vi "VIn SMU.vi"(8 "error in (no error)":errorcluster, 11 "Configuration":T2={"IVI Refnum in"="SMU4145", "Vin SMU Channel"="", "Voltage Level"=0.0, "Current Limit"=0.0}) -> (0 "error out":errorcluster, 3 "Measurements":T1)   [LabVIEW 2021]
uses:
  <instrlib>/niDCPower/nidcpower.llb/niDCPower Source Mode.ctl
  <instrlib>/niDCPower/nidcpower.llb/niDCPower Output Function.ctl
  controls/Current Meas.ctl
  controls/Data Holder.ctl
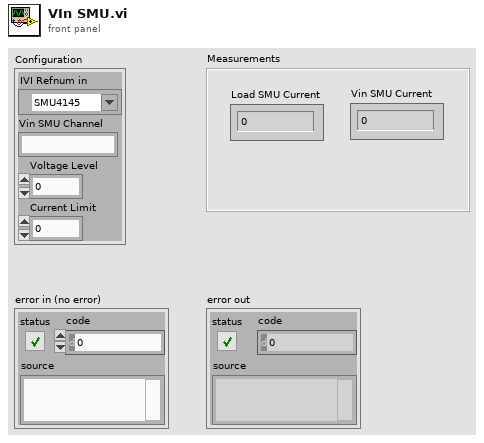
[diagram p1: front panel]
types:
  T1 = typedef "Current Meas.ctl" = cluster{"Load SMU Current":dbl, "Current Measurement":dbl}
  T2 = typedef "Data Holder.ctl" = cluster{"IVI Refnum in":refnum<k15>, "Vin SMU Channel":string, "Voltage Level":dbl, "Current Limit":dbl}
  T3 = typedef "niDCPower Output Function.ctl" = i32
  T4 = typedef "niDCPower Source Mode.ctl" = i32
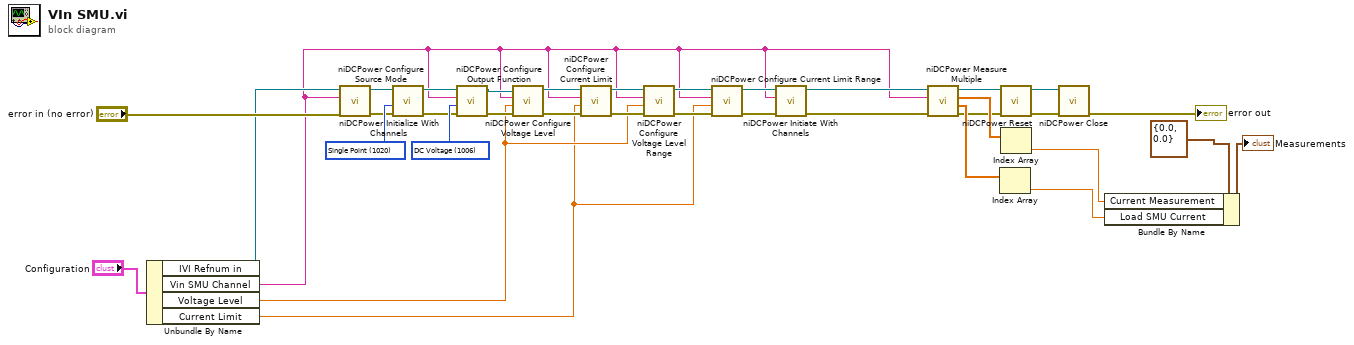
[diagram p0: block diagram]
diagram:
  w31 = T3 1006 items=["DC Voltage"=1006, "DC Current"=1007, "Pulse Voltage"=1049, "Pulse Current"=1050] ("output function")
  w18 = T4 1020 items=["Single Point"=1020, "Sequence"=1021] ("source mode")
  n1 = Unbundle By Name("Configuration") -> ("IVI Refnum in"=w8:refnum<k15>, "Vin SMU Channel"=w7:string, "Voltage Level"=w6:dbl, "Current Limit"=w5:dbl)
  n2 = call <instrlib>:"niDCPower Initialize With Channels.vi"("error in (no error)"="error in (no error)", "channels"=w7, "resource name"=w8) -> ("error out"=w14:errorcluster, "instrument handle out"=w15:refnum<k15>)  [unwired: 2 in, 5 out]
  n3 = call <instrlib>:"niDCPower Configure Source Mode.vi"("error in (no error)"=w14, "source mode"=w18, "instrument handle"=w15) -> ("error out"=w16:errorcluster, "instrument handle out"=w17:refnum<k15>)  [unwired: 7 out]
  n4 = call <instrlib>:"niDCPower Configure Output Function.vi"("error in (no error)"=w16, "output function"=w31, "channel name"=w7, "instrument handle"=w17) -> ("error out"=w30:errorcluster, "instrument handle out"=w29:refnum<k15>)  [unwired: 6 out]
  n5 = call <instrlib>:"niDCPower Configure Voltage Level.vi"("error in (no error)"=w30, "voltage level"=w6, "channel name"=w7, "instrument handle"=w29) -> ("error out"=w11:errorcluster, "instrument handle out"=w10:refnum<k15>)  [unwired: 6 out]
  n6 = call <instrlib>:"niDCPower Configure Current Limit.vi"("error in (no error)"=w11, "current limit"=w5, "channel name"=w7, "instrument handle"=w10) -> ("error out"=w19:errorcluster, "instrument handle out"=w20:refnum<k15>)  [unwired: 1 in, 5 out]
  n7 = call <instrlib>:"niDCPower Configure Voltage Level Range.vi"("error in (no error)"=w19, "voltage level range"=w6, "channel name"=w7, "instrument handle"=w20) -> ("error out"=w21:errorcluster, "instrument handle out"=w22:refnum<k15>)  [unwired: 6 out]
  n8 = call <instrlib>:"niDCPower Configure Current Limit Range.vi"("error in (no error)"=w21, "current limit range"=w5, "channel name"=w7, "instrument handle"=w22) -> ("error out"=w26:errorcluster, "instrument handle out"=w25:refnum<k15>)  [unwired: 6 out]
  n9 = call <instrlib>:"niDCPower Initiate With Channels.vi"("error in (no error)"=w26, "channel name"=w7, "instrument handle"=w25) -> ("error out"=w28:errorcluster, "instrument handle out"=w27:refnum<k15>)  [unwired: 7 in]
  n10 = call <instrlib>:"niDCPower Measure Multiple.vi"("error in (no error)"=w28, "channel name"=w7, "instrument handle"=w27) -> ("error out"=w24:errorcluster, "current measurements"=w33:dbl[], "voltage measurements"=w34:dbl[], "instrument handle out"=w23:refnum<k15>)  [unwired: 5 out]
  n11 = Index Array(array=w33) -> (element=w2:dbl)  [unwired: 1 in]
  n12 = call <instrlib>:"niDCPower Reset.vi"("error in (no error)"=w24, "instrument handle"=w23) -> ("error out"=w13:errorcluster, "instrument handle out"=w12:refnum<k15>)  [unwired: 2 in, 6 out]
  n13 = Index Array(array=w34) -> (element=w1:dbl)  [unwired: 1 in]
  n14 = call <instrlib>:"niDCPower Close.vi"("error in (no error)"=w13, "instrument handle"=w12) -> ("error out"=→"error out":errorcluster)  [unwired: 9 out]
  n15 = Bundle By Name(cluster=T1 {"Load SMU Current"=0.0, "Current Measurement"=0.0} ("Current Measurement 2"), "Current Measurement"=w1, "Load SMU Current"=w2) -> (→"Measurements":T1)
